vi "main.vi"() -> ()   [LabVIEW 2010]
uses:
  common_typedefs/channels_cluster.ctl
  common_typedefs/clock_parameters_cluster.ctl
  scan_specification_cluster.ctl
  common_typedefs/DAC_voltage_cluster.ctl
  derived_values_cluster.ctl
  counter_cluster.ctl
  integration_cluster.ctl
  common_typedefs/DAC_values_cluster.ctl
  common_typedefs/DAC_channel_enable_cluster.ctl
  <vilib>/Platform/TimedLoop/XDataNode/XDataNode.xnode
  <vilib>/Platform/TimedLoop/XDataNode/timing_clust.ctl
  <vilib>/Platform/TimedLoop/XDataNode/nitl_modes.ctl
  <vilib>/Platform/TimedLoop/XDataNode/wakeup.ctl
  <vilib>/eio/EIONode/EIONode.xnode
  <vilib>/rvi/eio/nirviEIOImplementation/nirviEIOImplementation.xnode
  <vilib>/rvi/eio/common/nirviEmuClasses.ctl
  <vilib>/rvi/eio/common/nirviEmuTemplateMethod_noerrors.vi
  <vilib>/Platform/TimedLoop/XDataNode/XDNodeRunTimeDep.lvlib
panel:
  in  "sync minimum high":i16=1000
  out "PIXEL COUNTER":u64(graph)
  out "Loop time":u32=100
  out "finished?":bool
  out "no of correct transferred z tuples":u32
  out "z-points transfer corrupt?":bool
  out "transferred z/intensity tuples":u32
  in  "transfer z-points?":bool
  in  "invert channels":bool[](array[boolean])=[FALSE, FALSE]
  in  "enable fly-back reversion?":bool=TRUE
  out "pixels acquired":u64
  out "counter cluster out":T1
  out "derived values":T2
  out "acquire?":bool
  in  "ADC clock phase":u8=2
  out "DAC voltages":T3 {"ch6" max=4095 step=1; "ch5" max=4095 step=1; "ch4" max=4095 step=1; "ch3" max=4095 step=1; "ch2" max=4095 step=1; "ch1" max=4095 step=1; "ch0" max=4095 step=1}
  in  "scan specification":T4={"x amplitude"=1000, "x resolution (pixels)"=100, "x offset fly-forward (iterations)"=0, "x offset fly-back (iterations)"=0, "y resolution (nr. of lines)"=200, "y step size"=5, "iterations per pixel"=5, "number of frames"=-1, "y offset (pixels)"=0, "number of y-brake lines  (before y-fly-back)"=2, "number y-brake lines (after y-fly-back)"=2, "number of y-fly-back steps"=2, "lines per z step"=5, "number of z/intensity tuples"=200, "number of repetitions (volumes or planes)"=500, "z step size derived"=0, "choose the beginning of z scan"=FALSE, "number of frames (settings)"=0, "FPGA trajectory?"=FALSE}
  out "clock 1 state":bool
  out "clock 2 state":bool
  in  "clock 2 settings":T5
  in  "clock 1 settings":T5
  out "data read":T6
  in  "maximum bit depth":i8
  out "FIFO overflow":bool
  in  "scan":bool
  in  "stop":bool
  in  "wait for trigger?":bool
  in  "stop acquisition at\nFIFO overflow?":bool
  out "scanning?":bool
  in  "converter box version":i16=2 min=1 max=2
  # "Mirna: \niterations per pixel = (x scan segment fraction*fFPGA)/(x resolution*f resonance)\nfFPGA/f resonance = 5000 --assumes 8kHz resonance frequency\niterations per pixel=25"
  # "used to be 1000 (Mirna)"
  # "y settings:\ny resolution*y step size = 6553\nthis gives scan from -1 to 1V\ny resolution = 200\ny step size = 33\n\nz settings:\nto scan entire y profile \nnumber of z's has to be equal\ny resolution"
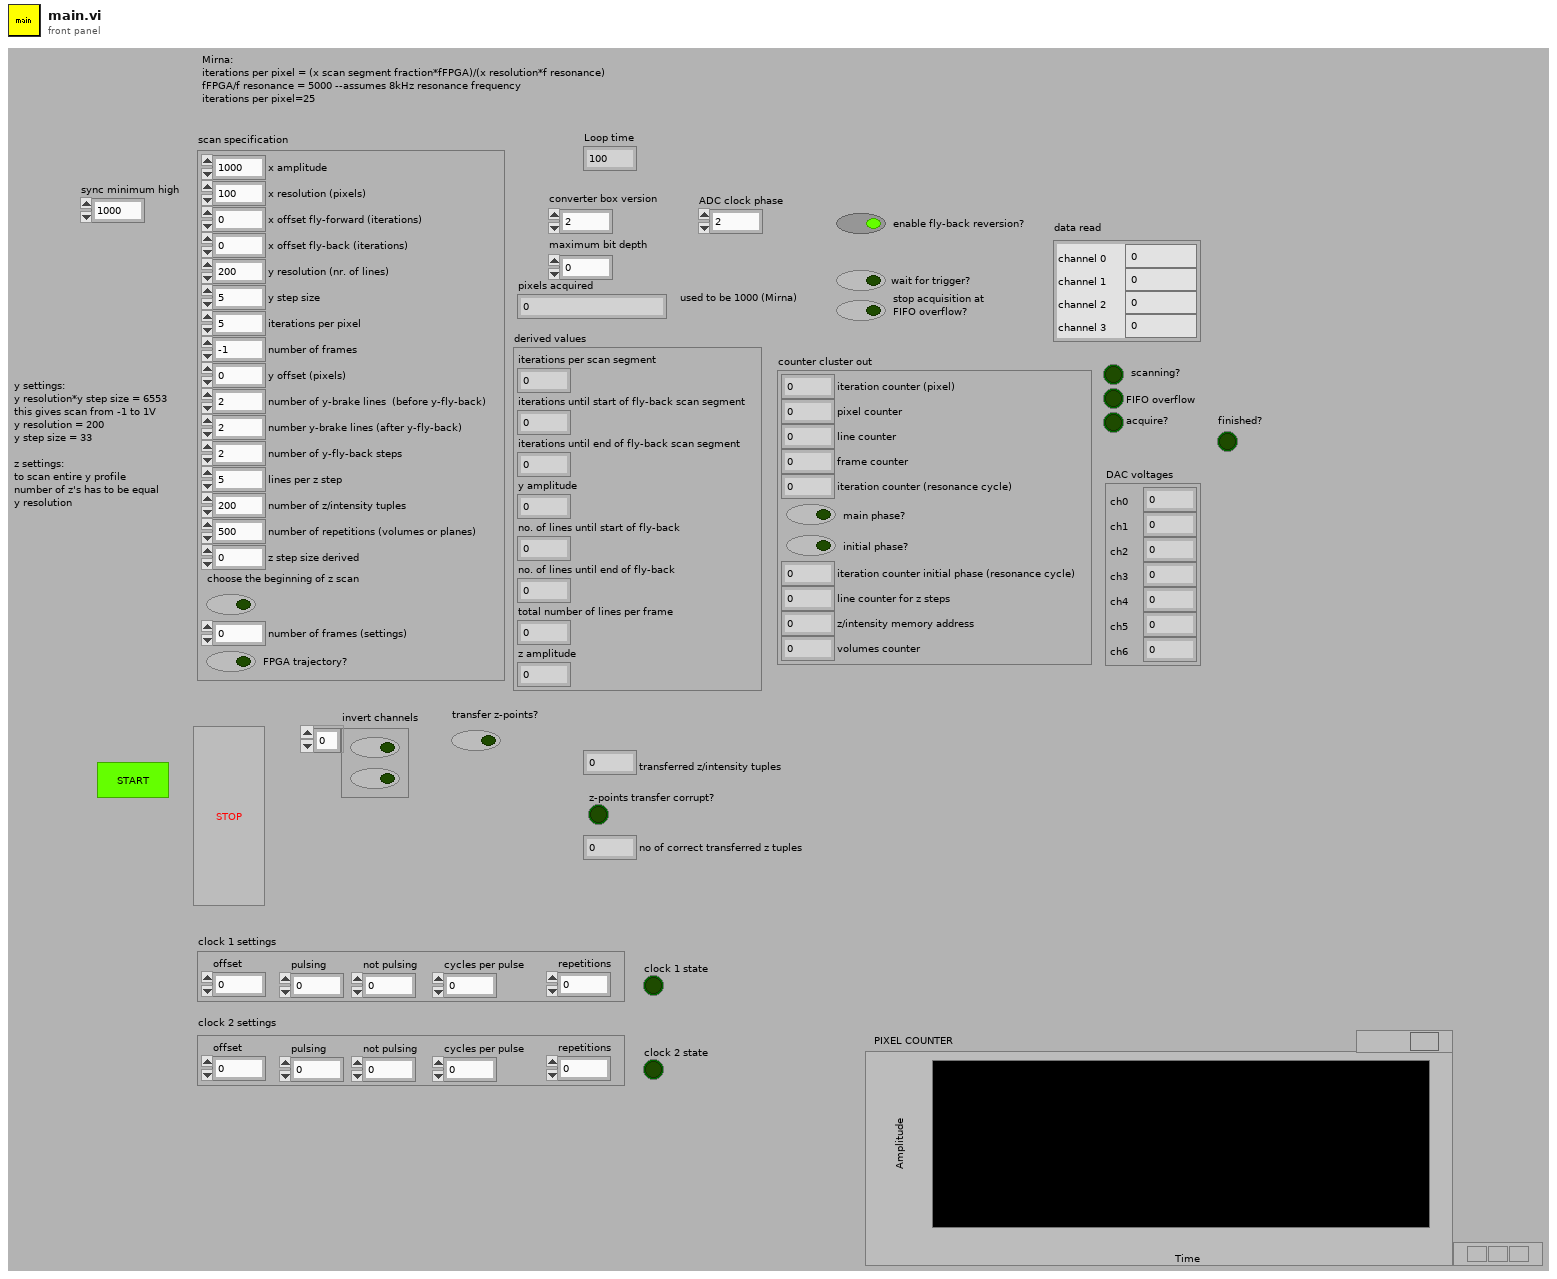
[diagram p1: front panel]
types:
  T1 = typedef "counter_cluster.ctl" = cluster{"iteration counter (pixel)":u16, "pixel counter":u16, "line counter":u16, "frame counter":u16, "iteration counter (resonance cycle)":u16, "main phase?":bool, "initial phase?":bool, "iteration counter initial phase (resonance cycle)":u16, "line counter for z steps":u16, "z/intensity memory address":u32, "volumes counter":u16}
  T2 = typedef "derived_values_cluster.ctl" = cluster{"iterations per scan segment":u16, "iterations until start of fly-back scan segment":u16, "iterations until end of fly-back scan segment":u16, "y amplitude":u16, "no. of lines until start of fly-back":u16, "no. of lines until end of fly-back":u16, "total number of lines per frame ":u16, "z amplitude":u16}
  T3 = typedef "DAC_voltage_cluster.ctl" = cluster{"ch0":u16, "ch1":i16, "ch2":i16, "ch3":u16, "ch4":u16, "ch5":u16, "ch6":u16}
  T4 = typedef "scan_specification_cluster.ctl" = cluster{"x amplitude":u16, "x resolution (pixels)":u16, "x offset fly-forward (iterations)":u16, "x offset fly-back (iterations)":u16, "y resolution (nr. of lines)":u16, "y step size":u16, "iterations per pixel":u16, "number of frames":i32, "y offset (pixels)":u16, "number of y-brake lines  (before y-fly-back)":u16, "number y-brake lines (after y-fly-back)":u16, "number of y-fly-back steps":u16, "lines per z step":u16, "number of z/intensity tuples":u16, "number of repetitions (volumes or planes)":i32, "z step size derived":u16, "choose the beginning of z scan":bool, "number of frames (settings)":i32, "FPGA trajectory?":bool}
  T5 = typedef "clock_parameters_cluster.ctl" = cluster{"offset":i64, "pulsing":i64, "not pulsing":i64, "cycles per pulse":i64, "repetitions":i64}
  T6 = typedef "channels_cluster.ctl" = cluster{"channel 0":u32, "channel 1":u32, "channel 2":u32, "channel 3":u32}
  T7 = typedef "DAC_values_cluster.ctl" = cluster{"DAC channel enable":T8, "DAC voltage":T3, "offset":u16, "channel index":u16, "bit index":i32, "synch?":bool, "DAC clock":bool, "finished?":bool}
  T8 = typedef "DAC_channel_enable_cluster.ctl" = cluster{"ch0":bool, "ch1":bool, "ch2":bool, "ch3":bool, "ch4":bool, "ch5":bool, "ch6":bool}
  T9 = typedef "integration_cluster.ctl" = cluster{"channel 0":u32, "channel 1":u32, "fly-back heap address":u32}
  T10 = typedef "XDNodeRunTimeDep.lvlib/timing_clust.ctl" = cluster{"Expected End [f-1]":u64, "Actual End [f-1]":u64, "Finished Late? [f-1]":bool, "Expected End [i-1]":u64, "Actual End [i-1]":u64, "Finished Late? [i-1]":bool, "Expected Start [i]":u64, "Actual Start [i]":u64, "Expected Start [f]":u64, "Actual Start [f]":u64, "Source Name":string, "Structure Name":string, "Period":i64, "Deadline":i64, "Offset":i64, "Start":i64, "Priority":i32, "Timeout":i32, "Mode":T11, "Wakeup Reason":T12, "Error":errorcluster, "Source Type":string, "Secondary Source Type":string, "Global End Time":u64, "Global Start Time":u64, "Frame Duration":u64, "Iteration Duration":u64, "Assigned CPU":i32, "I/O Scan Engine Mode":u32}
  T11 = typedef "XDNodeRunTimeDep.lvlib/nitl_modes.ctl" = enum32{"No Change", "Process missed periods, maintain original phase", "Discard missed periods, maintain original phase", "Process missed periods, ignore original phase", "Discard missed periods, ignore original phase"}
  T12 = typedef "XDNodeRunTimeDep.lvlib/wakeup.ctl" = enum32{"Normal", "Aborted", "Asynchronous wakeup", "Timing source error", "Timed loop error", "Timeout"}
  T13 = typedef "nirviEmuClasses.ctl" = enum16{"IO Read", "IO Write", "Method", "Property Read", "Property Write"}
  T14 = typedef "gate_counters_cluster.ctl" = cluster{"phase iteration counter":i64, "phase repetition counter":i64, "pulse iteration counter":i64, "phase state":bool}
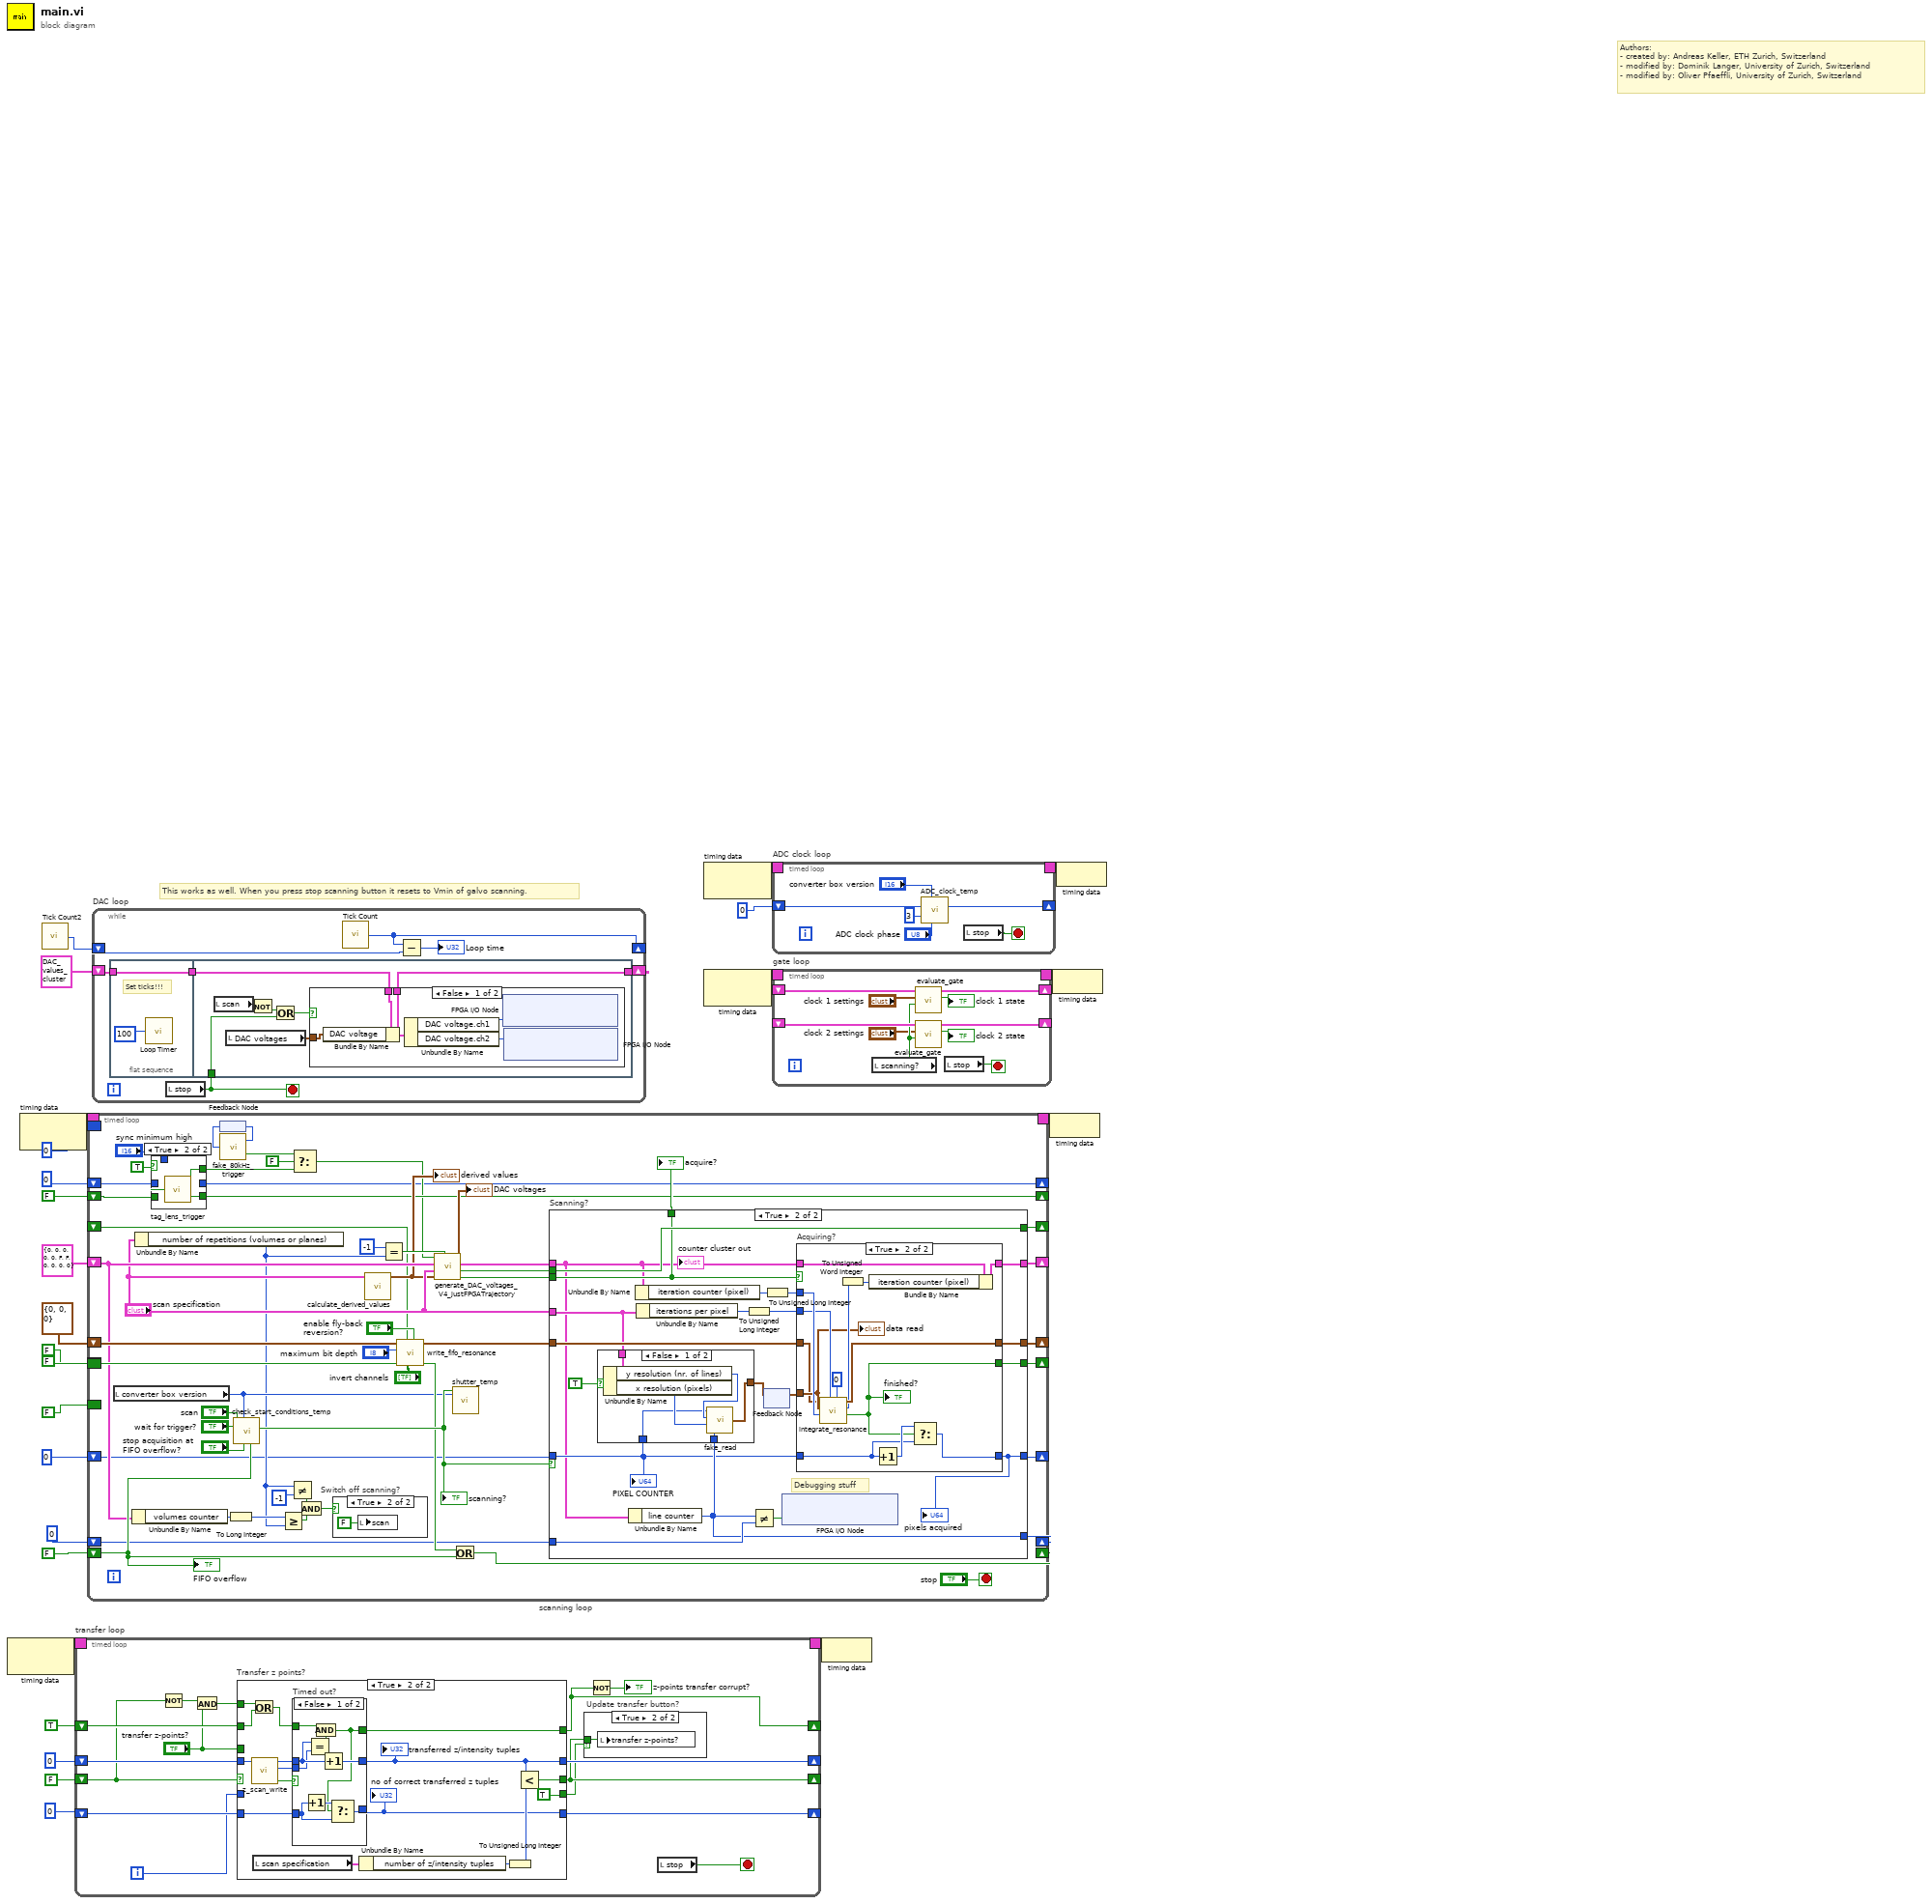
[diagram p0: block diagram]
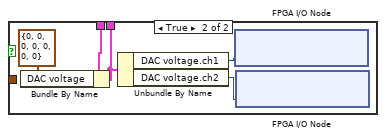
[diagram p2: hidden frame]
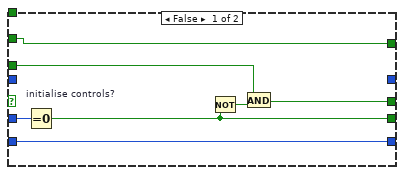
[diagram p4: hidden frame]
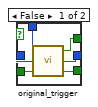
[diagram p6: hidden frame]
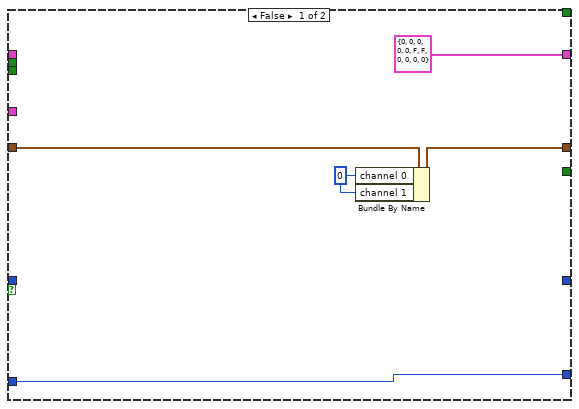
[diagram p8: hidden frame]
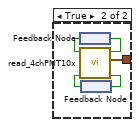
[diagram p9: hidden frame]
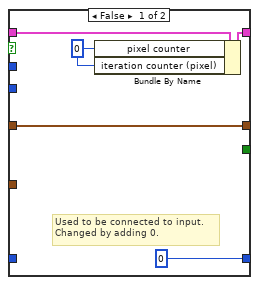
[diagram p10: hidden frame]
diagram:
  # "This works as well. When you press stop scanning button it resets to Vmin of galvo scanning."
  # "Authors: \n- created by: Andreas Keller, ETH Zurich, Switzerland\n- modified by: Dominik Langer, University of Zurich, Switzerland\n- modified by: Oliver Pfaeffli, University of Zurich, Switzerland"
  n1 = node-c288() -> (w11:T10)  [unwired: 1 in]
  n2 = node-c288() -> (w24:T10)  [unwired: 1 in]
  n3 = call "Tick Count2"() -> ("Tick Count(Ticks)"=w5:u32)
  n4 = timed-loop "transfer loop" {
    shift-right: [w40] -> _
    shift-left: u32 0 ("address out") -> [w41]
    timing: w11 -> [_]
    timing-out: [_] -> w10
    shift-right: [w32] -> _
    shift-left: FALSE ("start z-points transfer?") -> [w37]
    shift-right: [w38] -> _
    shift-left: TRUE ("start z-points transfer?") -> [w39]
    shift-right: [w35] -> _
    shift-left: u32 0 ("address out") -> [w36]
    i -> [w34]
    stop <- w33 stop-if-true
    n5 = Not(x=w37) -> (.not. x?=w29:bool)
    n6 = And(x=w29, y="transfer z-points?") -> (x .and. y?=w27:bool)
    n7 = case "Transfer z points?" shown="True" w37 {
      tunnel: w41 -> [_ w65]
      tunnel: [_ w63] -> w40
      tunnel: [w47 w59] -> w32
      tunnel: w34 -> [w49 _]
      tunnel: [w46 TRUE] -> w31
      tunnel: w39 -> [w45 w53]
      tunnel: [w45 w55] -> w38
      tunnel: "transfer z-points?" -> [w44 _]
      tunnel: w27 -> [_ w54]
      tunnel: w36 -> [w43 w51]
      tunnel: [w43 w50] -> w35
      frame False {
        n8 = Equal To 0? "initialise controls?"(x=w49) -> (x = 0?=w46:bool)
        n9 = Not(x=w46) -> (.not. x?=w48:bool)
        n10 = And(x=w44, y=w48) -> (x .and. y?=w47:bool)
      }
      frame True {
        n11 = Or(x=w54, y=w53) -> (x .or. y?=w52:bool)
        n12 = call "z_scan_write.vi"("address in"=w65) -> ("FIFO scan time out"=w57:bool, "data"=w56:u32, "address out"=w64:u32)  [unwired: 8 in]
        n13 = local read "scan specification"() -> (w62:T4)
        n14 = case "Timed out?" shown="False" w57 {
          tunnel: w64 -> [w71 w77]
          tunnel: [w74 w77] -> w63
          tunnel: w56 -> [w70 _]
          tunnel: w52 -> [w73 w76]
          tunnel: [w67 w76] -> w55
          tunnel: w51 -> [w69 w75]
          tunnel: [w66 w75] -> w50
          frame False {
            n15 = Increment(x=w69) -> (x+1=w68:u32)
            n16 = Equal?(x=w71, y=w70) -> (x = y?=w72:bool)
            n17 = And(x=w73, y=w72) -> (x .and. y?=w67:bool)
            n18 = Increment(x=w71) -> (x+1=w74:u32)
            n19 = Select(t=w68, s=w67, f=w69) -> (s? t:f=w66:u32)
          }
          frame True {
          }
        }
        "transferred z/intensity tuples" <- w63
        "no of correct transferred z tuples" <- w50
        n20 = Unbundle By Name(w62) -> ("number of z/intensity tuples"=w61:u16)
        n21 = To Unsigned Long Integer(number=w61) -> (unsigned 32bit integer=w60:u32)
        n22 = Less?(x=w63, y=w60) -> (x < y?=w59:bool)
      }
    }
    n23 = case "Update transfer button?" shown="True" w31 {
      tunnel: w32 -> [_ w42]
      frame False {
      }
      frame True {
        n24 = local write "transfer z-points?"(w42) -> ()
      }
    }
    n25 = Not(x=w38) -> (.not. x?=→"z-points transfer corrupt?":bool)
    n26 = local read "stop"() -> (w33:bool)
  }
  n27 = timed-loop "scanning loop" {
    timing: w24 -> [_]
    timing-out: [_] -> w23
    shift-right: [w130] -> _
    shift-left: T1 {"iteration counter (pixel)"=0, "pixel counter"=0, "line counter"=0, "frame counter"=0, "iteration counter (resonance cycle)"=0, "main phase?"=FALSE, "initial phase?"=FALSE, "iteration counter initial phase (resonance cycle)"=0, "line counter for z steps"=0, "z/intensity memory address"=0, "volumes counter"=0} ("counter cluster") -> [w109]
    shift-right: [w117] -> _
    shift-left: T9 {"channel 0"=0, "channel 1"=0, "fly-back heap address"=0} ("integration cluster") -> [w116]
    shift-right: [w119] -> _
    shift-left: FALSE -> [w111]
    shift-right: [w123] -> _
    shift-left: u64 0 -> [w81]
    shift-right: [w84] -> _
    shift-left: i16 0 -> [w85]
    shift-right: [w118] -> _
    shift-left: _ -> [w82]
    shift-right: [w113] -> _
    shift-left: FALSE ("finished?") -> [w112]
    shift-right: [w90] -> _
    shift-left: FALSE -> [w91]
    shift-right: [w94] -> _
    shift-left: u64 0 -> [w95]
    border: FALSE ("Inputl1") -> [_]
    border: FALSE ("Input0") -> [_]
    border: u16 0 -> [_]
    stop <- "stop" stop-if-true
    n28 = local read "converter box version"() -> (w101:i16)
    n29 = Unbundle By Name(w109) -> ("volumes counter"=w105:u16)
    n30 = Unbundle By Name("scan specification") -> ("number of repetitions (volumes or planes)"=w99:i32)
    n31 = case shown="True" TRUE {
      tunnel: w91 -> [w134 w139]
      tunnel: [w136 w141] -> w86
      tunnel: [w135 w140] -> w90
      tunnel: w85 -> [w138 _]
      tunnel: [w137 _] -> w84
      tunnel: "sync minimum high" -> [w133 _]
      frame False {
        n32 = call "original_trigger.vi"("last sync value"=w134, "counter in"=w138, "sync minimum high"=w133) -> ("DIO stored in shift registar"=w135:bool, "counter out"=w137:i16, "trigger out"=w136:bool)
      }
      frame True {
        n33 = call "tag_lens_trigger.vi"("previous DIO value"=w139) -> ("DIO to shift registar"=w140:bool, "trigger out"=w141:bool)
      }
    }
    n34 = feedback #1() -> (w100:u16)
    n35 = call "fake_80kHz_trigger.vi"("Counter in"=w100) -> ("trigger"=w87:bool, "Counter out"=w96:u16)
    n36 = feedback-in #1(w96) -> ()
    n37 = To Long Integer(number=w105) -> (32bit integer=w104:i32)
    n38 = call "check_start_conditions_temp.vi"("FIFO overflow?"=w111, "stop at FIFO overflow?"="stop acquisition at\nFIFO overflow?", "converter box version"=w101, "in triggered mode?"="wait for trigger?", "acquire"="scan") -> ("acquire?"=w125:bool)  [unwired: 6 in]
    "scanning?" <- w125
    n39 = Greater Or Equal?(x=w104, y=w99) -> (x >= y?=w127:bool)
    n40 = Not Equal?(x=w99, y=-1) -> (x != y?=w124:bool)
    n41 = Select(t=w87, s=FALSE, f=w86) -> (s? t:f=w89:bool)
    n42 = And(x=w124, y=w127) -> (x .and. y?=w97:bool)
    n43 = case "Switch off scanning?" shown="True" w97 {
      frame False {
      }
      frame True {
        n44 = local write "scan"(FALSE ("scan")) -> ()
      }
    }
    n45 = call "calculate_derived_values.vi"("scan specification"="scan specification") -> ("derived values"=w98:T2)  [unwired: 10 in]
    "derived values" <- w98
    n46 = Equal?(x=-1, y=w99) -> (x = y?=w102:bool)
    n47 = call "write_fifo_resonance.vi"("enable fly-back reversion?"="enable fly-back reversion?", "invert channels"="invert channels", "fly-back?"=w82, "pixel finished?"=w112, "maximum bit depth"="maximum bit depth", "integration cluster in"=w116) -> ("FIFO overflow out"=w114:bool, "integration cluster out"=w115:T9)  [unwired: 4 in]
    n48 = call "generate_DAC_voltages_V4_justFPGATrajectory.vi"("focus mode?"=w102, "derived values"=w98, "scan specification"="scan specification", "counter cluster in"=w109, "resonant trigger"=w89) -> ("acquire?"=w106:bool, "fly-back acquisition phase?"=w80:bool, "counter cluster out"=w108:T1, "DAC voltages"=→"DAC voltages":T3)  [unwired: 3 in]
    n49 = call "shutter_temp.vi"("converter box version"=w101, "open?"=w125) -> ()  [unwired: 10 in]
    n50 = Or(x=w114, y=w111) -> (x .or. y?=w119:bool)
    n51 = case "Scanning?" shown="True" w125 {
      tunnel: w108 -> [_ w148]
      tunnel: [T1 {"iteration counter (pixel)"=0, "pixel counter"=0, "line counter"=0, "frame counter"=0, "iteration counter (resonance cycle)"=0, "main phase?"=FALSE, "initial phase?"=FALSE, "iteration counter initial phase (resonance cycle)"=0, "line counter for z steps"=0, "z/intensity memory address"=0, "volumes counter"=0} ("counter cluster") w167] -> w130
      tunnel: w115 -> [w145 w163]
      tunnel: [w144 w166] -> w117
      tunnel: "scan specification" -> [_ w151]
      tunnel: w81 -> [_ w149]
      tunnel: [_ w160] -> w123
      tunnel: [_ w157] -> w122
      tunnel: [_ w159] -> w113
      tunnel: [_ w158] -> w118
      tunnel: w80 -> [_ w158]
      tunnel: w106 -> [_ w157]
      tunnel: [w143 w150] -> w94
      tunnel: w95 -> [w143 w156]
      frame False {
        w146 = u32 0 ("channel 0")
        n52 = Bundle By Name(cluster=w145, "channel 0"=w146, "channel 1"=w146) -> (w144:T9)
      }
      frame True {
        # "Debugging stuff"
        n53 = Unbundle By Name(w148) -> ("line counter"=w150:u16)
        n54 = case shown="False" TRUE {
          tunnel: [w173 w174] -> w153
          tunnel: w151 -> [w172 _]
          tunnel: w150 -> [w169 _]
          tunnel: w149 -> [w168 _]
          frame False {
            n55 = Unbundle By Name(w172) -> ("y resolution (nr. of lines)"=w171:u16, "x resolution (pixels)"=w170:u16)
            n56 = call "fake_read.vi"("line counter"=w169, "x resolution (pixels)"=w170, "y resolution (nr. of lines)"=w171, "Numeric"=w168) -> ("input cluster"=w173:T6)
          }
          frame True {
            n57 = feedback #2() -> (w175:bool)
            n58 = feedback #3() -> (w177:bool)
            n59 = call "read_4chPMT10x.vi"("previous value ch1"=w177, "previous value ch0"=w175) -> ("Inputl1"=w176:bool, "read output"=w174:T6, "Input0"=w178:bool)  [unwired: 7 in]
            n60 = feedback-in #2(w178) -> ()
            n61 = feedback-in #3(w176) -> ()
          }
        }
        n62 = Unbundle By Name(w148) -> ("iteration counter (pixel)"=w165:u16)
        n63 = Unbundle By Name(w151) -> ("iterations per pixel"=w164:u16)
        n64 = To Unsigned Long Integer(number=w164) -> (unsigned 32bit integer=w161:u32)
        n65 = Not Equal?(x=w150, y=w156) -> (x != y?=w155:bool)
        n66 = To Unsigned Long Integer(number=w165) -> (unsigned 32bit integer=w162:u32)
        n67 = feedback #4() -> (w154:T6)  [unwired: 1 in]
        n68 = feedback-in #4(w153) -> ()
        n69 = xnode "FPGA I/O Node"("Connector0/DIO0"=w155) -> ()  [unwired: 1 in, 1 out]
        n70 = case "Acquiring?" shown="True" w157 {
          tunnel: w148 -> [w193 w203]
          tunnel: [w194 w201] -> w167
          tunnel: [w191 w206] -> w166
          tunnel: w163 -> [w191 w199]
          tunnel: w162 -> [_ w207]
          tunnel: w154 -> [_ w202]
          tunnel: w161 -> [_ w204]
          tunnel: w149 -> [_ w196]
          tunnel: [u64 0 w198] -> w160
          tunnel: [_ w195] -> w159
          frame False {
            w192 = u16 0 ("pixel counter")
            # "Used to be connected to input.\nChanged by adding 0."
            n71 = Bundle By Name(cluster=w193, "pixel counter"=w192, "iteration counter (pixel)"=w192) -> (w194:T1)
          }
          frame True {
            n72 = call "integrate_resonance.vi"("waiting iterations per pixel"=u32 0, "integration iterations per pixel"=w204, "iteration counter in"=w207, "sampling values in"=w202, "integration cluster in"=w199) -> ("finished?"=w195:bool, "iteration counter out"=w205:u32, "integration cluster out"=w206:T9)  [unwired: 4 in]
            "finished?" <- w195
            n73 = To Unsigned Word Integer(number=w205) -> (unsigned 16bit integer=w208:u16)
            n74 = Bundle By Name(cluster=w203, "iteration counter (pixel)"=w208) -> (w201:T1)
            n75 = Increment(x=w196) -> (x+1=w197:u64)
            n76 = Select(t=w197, s=w195, f=w196) -> (s? t:f=w198:u64)
            "data read" <- w202
          }
        }
        "pixels acquired" <- w160
        "counter cluster out" <- w148
        "PIXEL COUNTER" <- w149
      }
    }
    "acquire?" <- w122
    "FIFO overflow" <- w111
  }
  n77 = while "DAC loop" {
    shift-right: [w217] -> _
    shift-left: T7 {"DAC channel enable"={"ch0"=FALSE, "ch1"=FALSE, "ch2"=FALSE, "ch3"=FALSE, "ch4"=FALSE, "ch5"=FALSE, "ch6"=FALSE}, "DAC voltage"={"ch0"=0, "ch1"=0, "ch2"=0, "ch3"=0, "ch4"=0, "ch5"=0, "ch6"=0}, "offset"=0, "channel index"=0, "bit index"=0, "synch?"=FALSE, "DAC clock"=FALSE, "finished?"=FALSE} ("DAQ values out") -> [w216]
    shift-right: [w214] -> _
    shift-left: w5 -> [w213]
    stop <- w211 stop-if-true
    n78 = flat-sequence {
      tunnel: w216 -> [w219]
      tunnel: [w219] -> w215
      tunnel: [w226] -> w217
      tunnel: w215 -> [w225]
      tunnel: w211 -> [w224]
      frame #0 {
        # "Set ticks!!!"
        n79 = call "Loop Timer"("Count(Ticks)"=u32 100) -> ()  [unwired: 1 out]
      }
      frame #1 {
        n80 = local read "scan"() -> (w221:bool)
        n81 = local read "DAC voltages"() -> (w220:T3)
        n82 = Not(x=w221) -> (.not. x?=w222:bool)
        n83 = Or(x=w222, y=w224) -> (x .or. y?=w223:bool)
        n84 = case shown="False" w223 {
          tunnel: w220 -> [w229 _]
          tunnel: w225 -> [w228 w257]
          tunnel: [w227 w254] -> w226
          frame False {
            n85 = Bundle By Name(cluster=w228, "DAC voltage"=w229) -> (w227:T7)
            n86 = Unbundle By Name(w227) -> ("DAC voltage.ch1"=w230:i16, "DAC voltage.ch2"=w231:i16)
            n87 = xnode "FPGA I/O Node"("Connector0/AO0"=w230) -> ()  [unwired: 1 in, 1 out]
            n88 = xnode "FPGA I/O Node"("Connector0/AO1"=w231) -> ()  [unwired: 1 in, 1 out]
          }
          frame True {
            n89 = Bundle By Name(cluster=w257, "DAC voltage"=T3 {"ch0"=0, "ch1"=0, "ch2"=0, "ch3"=0, "ch4"=0, "ch5"=0, "ch6"=0}) -> (w254:T7)
            n90 = Unbundle By Name(w254) -> ("DAC voltage.ch1"=w255:i16, "DAC voltage.ch2"=w256:i16)
            n91 = xnode "FPGA I/O Node"("Connector0/AO0"=w255) -> ()  [unwired: 1 in, 1 out]
            n92 = xnode "FPGA I/O Node"("Connector0/AO1"=w256) -> ()  [unwired: 1 in, 1 out]
          }
        }
      }
    }
    n93 = local read "stop"() -> (w211:bool)
    n94 = call "Tick Count"() -> ("Tick Count(Ticks)"=w214:u32)
    n95 = Subtract(x=w214, y=w213) -> (x-y=→"Loop time":u32)
  }
  n96 = node-c288() -> (w15:T10)  [unwired: 1 out]
  n97 = node-c288() -> (w26:T10)  [unwired: 1 in]
  n98 = timed-loop "ADC clock loop" {
    timing: w15 -> [_]
    timing-out: [_] -> w14
    shift-right: [w283] -> _
    shift-left: u8 0 -> [w284]
    stop <- w286 stop-if-true
    n99 = call "ADC_clock_temp.vi"("phase"="ADC clock phase", "converter box version"="converter box version", "iterations per cycle"=u8 3, "counter in"=w284) -> ("counter out"=w283:u8)  [unwired: 7 in]
    n100 = local read "stop"() -> (w286:bool)
  }
  n101 = timed-loop "gate loop" {
    timing: w26 -> [_]
    timing-out: [_] -> w25
    shift-right: [w297] -> _
    shift-left: _ -> [w298]
    shift-right: [w295] -> _
    shift-left: _ -> [w294]
    stop <- w296 stop-if-true
    n102 = local read "scanning?"() -> (w293:bool)
    n103 = call "evaluate_gate.vi"("acquiring?"=w293, "gate settings"="clock 1 settings", "gate counters in"=w298) -> ("pulse state out"=→"clock 1 state":bool, "gate counters out"=w297:T14)  [unwired: 7 in]
    n104 = call "evaluate_gate.vi"("acquiring?"=w293, "gate settings"="clock 2 settings", "gate counters in"=w294) -> ("pulse state out"=→"clock 2 state":bool, "gate counters out"=w295:T14)  [unwired: 7 in]
    n105 = local read "stop"() -> (w296:bool)
  }
  n106 = node-c288(w10) -> ()
  n107 = node-c288(w23) -> ()
  n108 = node-c288(w25) -> ()
  n109 = node-c288(w14) -> ()
